vi "Convert_String_to_TimeStamp.vi"(1 "date/time string":string) -> (0 "Resulting Time Stamp":timestamp format="%<%x>T")   [LabVIEW 2012]
doc: "This VI convert a date/time string back to a time stamp."
panel:
  # "This control should have data in the form:\n4/30/2004"
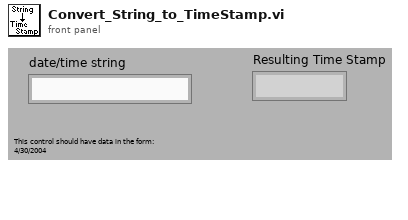
[diagram p1: front panel]
types:
  T1 = cluster{"second":i32, "minute":i32, "hour":i32, "day of month":i32, "month":i32, "year":i32, "day of week":i32, "day of year":i32, "is DST":i32}
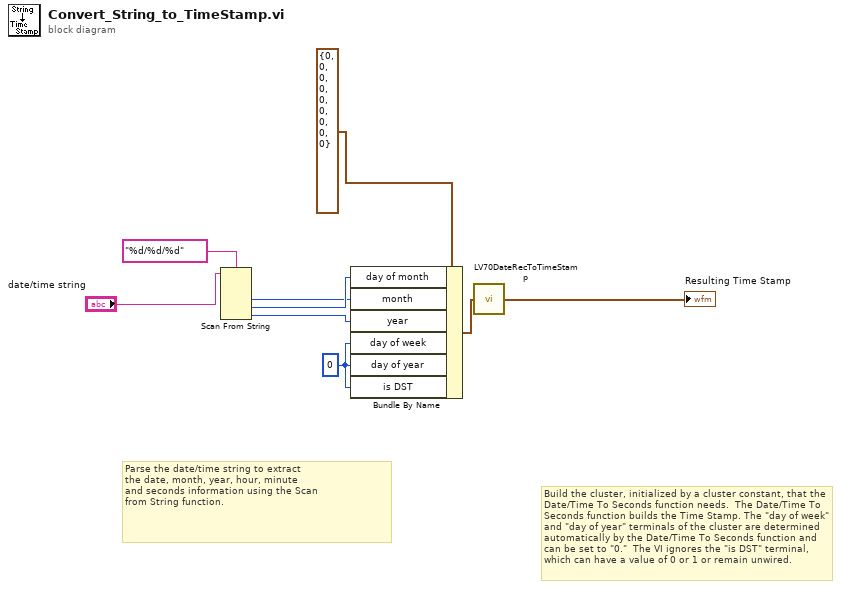
[diagram p0: block diagram]
diagram:
  w4 = 0
  # "Build the cluster, initialized by a cluster constant, that the Date/Time To Seconds function needs.  The Date/Time To Seconds function builds the Time Stamp. The \"day of week\" and \"day of year\" terminals of the cluster are determined automatically by the Date/Time To Seconds function and can be set to \"0.\"  The VI ignores the \"is DST\" terminal, which can have a value of 0 or 1 or remain unwired."
  # "Parse the date/time string to extract \nthe date, month, year, hour, minute \nand seconds information using the Scan\nfrom String function."
  n1 = Scan From String "Scan From String"(format string="%d/%d/%d", input string="date/time string") -> (output 1=w2:i32, output 2=w3:i32, output 3=w1:i32)  [unwired: 5 in, 3 out]
  n2 = Bundle By Name(cluster=T1 {"second"=0, "minute"=0, "hour"=0, "day of month"=0, "month"=0, "year"=0, "day of week"=0, "day of year"=0, "is DST"=0} ("date time rec"), "day of month"=w3, "month"=w2, "year"=w1, "day of week"=w4, "day of year"=w4, "is DST"=w4) -> (w5:T1)
  n3 = call <vilib>:"LV70DateRecToTimeStamp.vi"("date time rec"=w5) -> ("Time Stamp"=→"Resulting Time Stamp":timestamp)
